vi "Divisor_Sum_Engine.vi"(11 "N":i32) -> (2 "Numeric":i32, 3 "Array":i32[](array[numeric]))   [LabVIEW 2026]
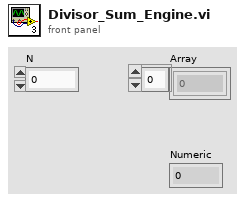
[diagram p1: front panel]
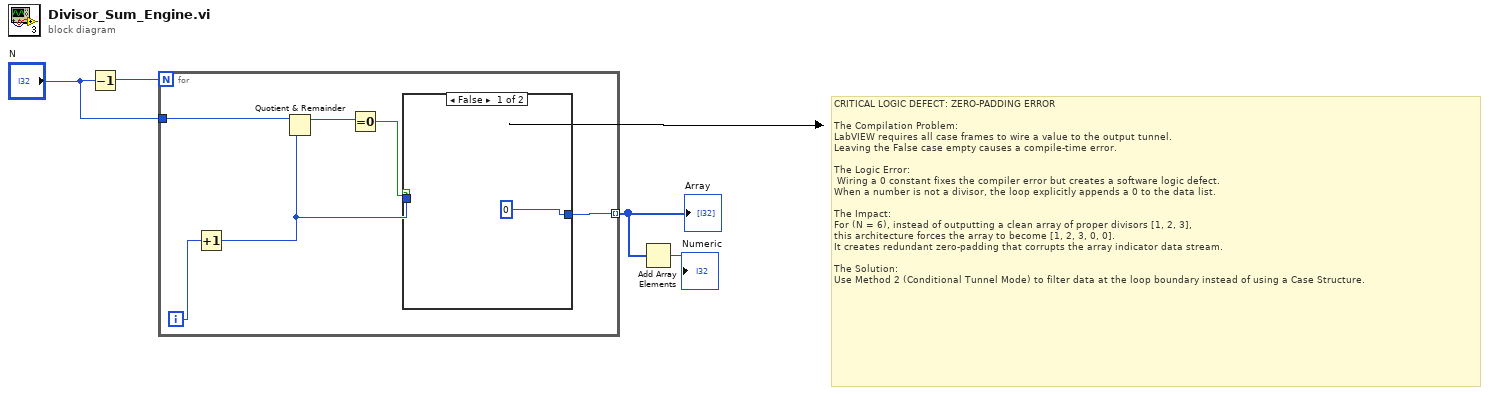
[diagram p0: block diagram]
diagram:
  # "CRITICAL LOGIC DEFECT: ZERO-PADDING ERROR \n\nThe Compilation Problem: \nLabVIEW requires all case frames to wire a value to the output tunnel. \nLeaving the False case empty causes a compile-time error.\n\nThe Logic Error:\n Wiring a 0 constant fixes the compiler error but creates a software logic defect. \nWhen a number is not a divisor, the loop explicitly appends a 0 to the data list.\n\nThe Impact: \nFor (N = 6), instead of outputting a clean array of proper divisors [1, 2, 3], \nthis architecture forces the array to become [1, 2, 3, 0, 0]. \nIt creates redundant zero-padding that corrupts the array indicator data stream.\n\nThe Solution: \nUse Method 2 (Conditional Tunnel Mode) to filter data at the loop boundary instead of using a Case Structure."
  n1 = Decrement(x="N") -> (x-1=w1:i32)
  n2 = for {
    N: w1 -> [_]
    tunnel: "N" -> [w9]
    tunnel: [w5] -> w3 mode=indexing
    i -> [w10]
    n3 = Increment(x=w10) -> (x+1=w6:i32)
    n4 = Quotient & Remainder(x=w9, y=w6) -> (x-y*floor(x/y)=w8:i32)  [unwired: 1 out]
    n5 = Equal To 0?(x=w8) -> (x = 0?=w7:bool)
    n6 = case shown="False" w7 {
      tunnel: [0 w12] -> w5
      tunnel: w6 -> [_ w12]
      frame False {
      }
      frame True {
      }
    }
  }
  "Array" <- w3
  n7 = Add Array Elements(numeric array=w3) -> (sum=→"Numeric":i32)
